vi "test EDS Viewer.vi"() -> ()   [LabVIEW 2024]
uses:
  EDS Viewer.lvclass
  C:/Program Files/National Instruments/LabVIEW 2024/vi.lib/MGI/Panel Manager/Panel Actor/Panel Actor/Panel Actor.lvclass
  <vilib>/ActorFramework/Message Enqueuer/Message Enqueuer.lvclass/Message Enqueuer.ctl
  <vilib>/ActorFramework/Message Enqueuer/Enqueue.vi
  EDS Viewer Messages/Populate Tree Items Msg/Populate Tree Items Msg.lvclass
  C:/Program Files/National Instruments/LabVIEW 2024/vi.lib/ActorFramework/Message/Message.lvclass
  <vilib>/MGI/Panel Manager/Panel Actor/Panel Actor/Launch Root Panel Window.vi
  <vilib>/Utility/LVClass/Get LV Class Name.vi
  <resource>/AFDebug/Generate Trace for Message.vi
  <vilib>/ActorFramework/Message Priority Queue/Priority Enqueue.vi
  <vilib>/MGI/Panel Manager/Panel Actor/Panel Actor/Panel Actor.lvclass
  C:/Program Files/National Instruments/LabVIEW 2024/vi.lib/ActorFramework/Actor/Actor.lvclass
  D:/git/CANopen-XNET/EDS Viewer/EDS Viewer/EDS Viewer.lvclass
panel:
  out "error out":errorcluster
  in  "File Path":path=path "D:/git/CANopen-XNET/EDS Viewer/C5-E-2-09.eds"
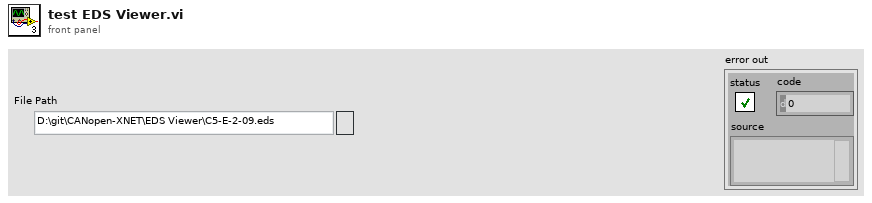
[diagram p1: front panel]
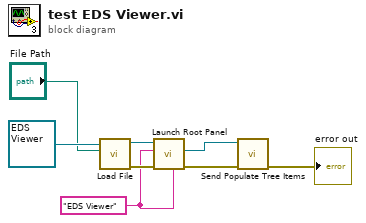
[diagram p0: block diagram]
diagram:
  w4 = "EDS Viewer" ("Title")
  n1 = call-dynamic "Load File.vi"("File Path"="File Path", "EDS Viewer in"=refnum<class "EDS Viewer.lvclass"> refnum ("EDS Viewer.lvlib:EDS Viewer.lvclass")) -> ("error out"=w6:errorcluster, "EDS Viewer out"=w5:refnum<class "EDS Viewer.lvclass">)  [unwired: 8 in]
  n2 = call-poly <vilib>:"Launch Root Panel.vi"("Debug Alias"=w4, "Error In"=w6, "Title"=w4, "Panel Actor in"=w5) -> ("Error Out"=w2:errorcluster, "Actor's Enqueuer"=w3:refnum<class "Message Enqueuer.lvclass">)  [unwired: 6 in]
  n3 = call "Send Populate Tree Items.vi"("error in (no error)"=w2, "Message Enqueuer"=w3) -> ("error out"=→"error out":errorcluster)  [unwired: 8 in, 1 out]
